vi "Show Values Graphs.vi"() -> ()   [LabVIEW 2014]
uses:
  <vilib>/Native 3D Graph/xcontrol/3DPC_SurfacePlot.xctl
panel:
  out "3D Graph":refnum<class "Base Datatype.lvclass">[](xcontrol)
  out "Waveform Chart":cluster{dbl, dbl, dbl}(graph)
  out "read buffer":string
  out "error out":errorcluster
  in  "stop":bool
  in  "error in":errorcluster
  in  "Serial port":refnum<visa-resource-name>
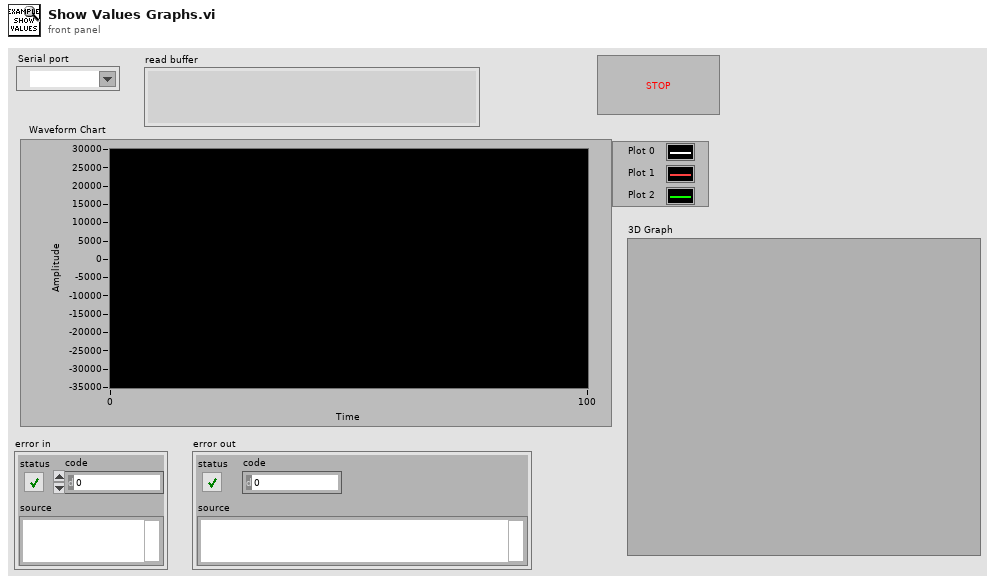
[diagram p1: front panel]
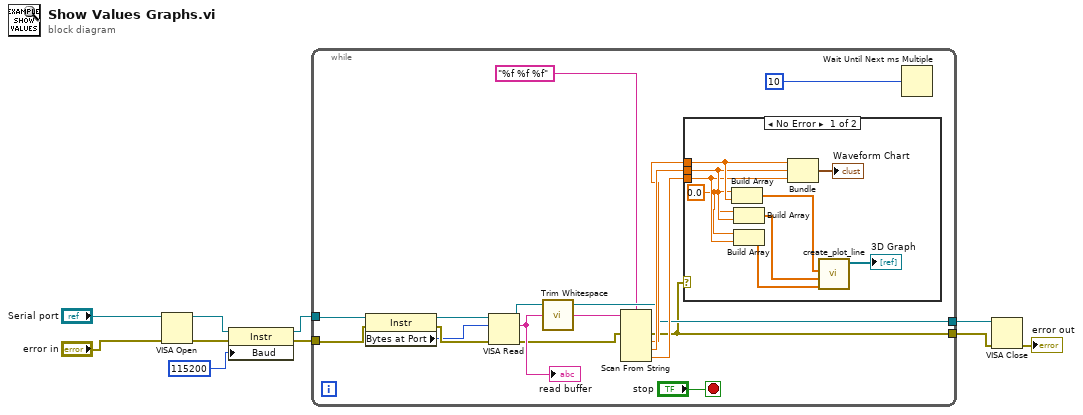
[diagram p0: block diagram]
diagram:
  n1 = VISA Open(error in (no error)="error in", VISA resource name="Serial port") -> (VISA resource name=w8:refnum<visa-resource-name>, error out=w6:errorcluster)  [unwired: 3 in]
  n2 = property class="Instr"(reference=w8, error in=w6, "Baud"=u32 115200 ("Serial Settings:Baud Rate")) -> (reference out=w7:refnum<visa-resource-name>, error out=w5:errorcluster)
  n3 = while {
    tunnel: w7 -> [w26]
    tunnel: w5 -> [w17]
    tunnel: [w13] -> w3
    tunnel: [w19] -> w2
    stop <- "stop" stop-if-true
    n4 = property class="Instr"(reference=w26, error in=w17) -> (reference out=w18:refnum<visa-resource-name>, error out=w16:errorcluster, "Bytes at Port"=w15:u32)
    n5 = VISA Read(VISA resource name=w18, byte count=w15, error in (no error)=w16) -> (VISA resource name out=w19:refnum<visa-resource-name>, read buffer=w24:string, error out=w20:errorcluster)  [unwired: 1 out]
    "read buffer" <- w24
    n6 = call <vilib>:"Trim Whitespace.vi"("string"=w24) -> ("trimmed string"=w11:string)  [unwired: 1 in]
    n7 = Scan From String(format string="%f %f %f", input string=w11, error in=w20) -> (error out=w13:errorcluster, output 1=w21:dbl, output 2=w22:dbl, output 3=w23:dbl)  [unwired: 4 in, 2 out]
    n8 = case shown="No Error" w13 {
      tunnel: w23 -> [w31 _]
      tunnel: w22 -> [w32 _]
      tunnel: w21 -> [w33 _]
      frame No Error {
        w30 = 0.0 ("element")
        n9 = Build Array(w30, w33) -> (w29:dbl[])
        n10 = Build Array(w30, w32) -> (w28:dbl[])
        n11 = Build Array(w30, w31) -> (w27:dbl[])
        n12 = Bundle(w33, w32, w31) -> (→"Waveform Chart":cluster{dbl, dbl, dbl})  [unwired: 1 in]
        n13 = call <vilib>:"create_plot_line.vi"("z vector"=w27, "y vector"=w28, "x vector"=w29) -> ("plots out"=→"3D Graph":refnum<class "Base Datatype.lvclass">[])  [unwired: 2 in, 6 out]
      }
      frame Error {
      }
    }
    n14 = Wait Until Next ms Multiple(millisecond multiple=u32 10) -> ()  [unwired: 1 out]
  }
  n15 = VISA Close(VISA resource name=w2, error in (no error)=w3) -> (error out=→"error out":errorcluster)
